vi "cDAQ_PLC.vi"(6 "simulazione":bool, 9 "banco":i32, 11 "carico res":bool=TRUE) -> ()   [LabVIEW 2019]
uses:
  controls/statoDO_Cdaq.ctl
  controls/StatoAO_cdaq.ctl
  cDAQ/SET SINGLE DO.ctl
  cDAQ/DO List.ctl
  cDAQ/SET ARRAY AO.ctl
  cDAQ/SET SINGLE AO.ctl
  cDAQ/AO List.ctl
  TypeDef/Lista AO sistema.ctl
  TypeDef/DOinterfaccia.ctl
  ST1200_LIST_IO/StatoDO_PLC_1.ctl
  ST1200_LIST_IO/StatoDO_PLC_2.ctl
  ST1200_LIST_IO/StatoDO_PLC_3.ctl
  controls/statoAO_plc_1.ctl
  controls/statoAO_plc_2.ctl
  controls/statoAO_plc_3.ctl
  ST1200_LIST_IO/TypeDef_PLC_Q.ctl
  ST1200_LIST_IO/Uscite PLC 2.ctl
  ST1200_LIST_IO/Uscite PLC 3.ctl
  EXIT.vi
  <vilib>/Utility/file.llb/Read Delimited Spreadsheet (string).vi
  Global dati targa SINUSPENTA.vi
panel:
  out "AO Tread ms":u32
  out "DO Tread ms":u32
  out "statoAO_Cdaq out":T1
  out "elements in queue AO":i32
  out "statoDO Cdaq out":T2
  out "elements in queue DO":i32
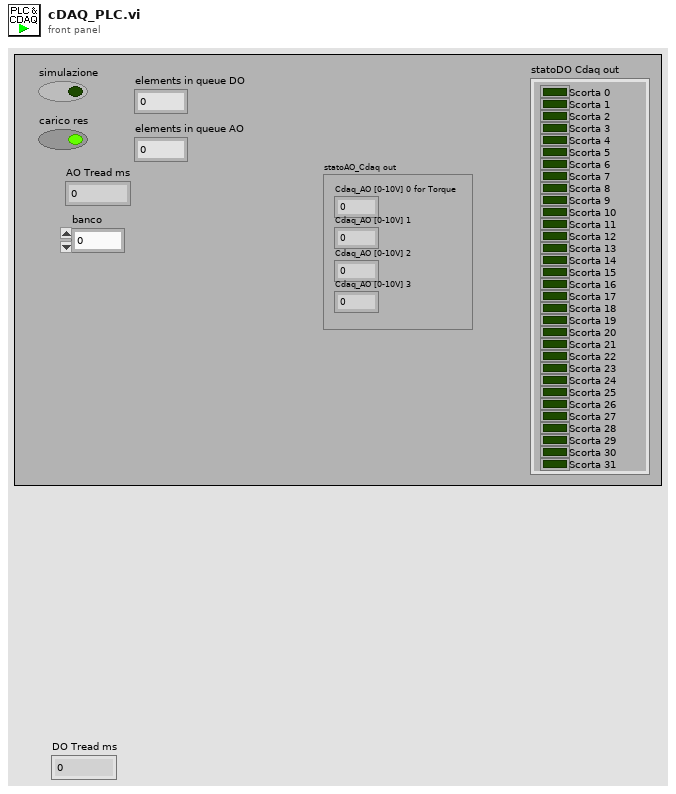
[diagram p1: front panel]
types:
  T1 = typedef "StatoAO_cdaq.ctl" = cluster{"Cdaq_AO [0-10V] 0 for Torque":dbl, "Cdaq_AO [0-10V] 1":dbl, "Cdaq_AO [0-10V] 2":dbl, "Cdaq_AO [0-10V] 3":dbl}
  T2 = typedef "statoDO_Cdaq.ctl" = cluster{"Scorta 0":bool, "Scorta 1":bool, "Scorta 2":bool, "Scorta 3":bool, "Scorta 4":bool, "Scorta 5":bool, "Scorta 6":bool, "Scorta 7":bool, "Scorta 8":bool, "Scorta 9":bool, "Scorta 10":bool, "Scorta 11":bool, "Scorta 12":bool, "Scorta 13":bool, "Scorta 14":bool, "Scorta 15":bool, "Scorta 16":bool, "Scorta 17":bool, "Scorta 18":bool, "Scorta 19":bool, "Scorta 20":bool, "Scorta 21":bool, "Scorta 22":bool, "Scorta 23":bool, "Scorta 24":bool, "Scorta 25":bool, "Scorta 26":bool, "Scorta 27":bool, "Scorta 28":bool, "Scorta 29":bool, "Scorta 30":bool, "Scorta 31":bool}
  T3 = typedef "TypeDef_PLC_Q.ctl" = cluster{"Message":string, "Data":variant}
  T4 = typedef "statoAO_plc_1.ctl" = cluster{"Rif Lim coppia freno [%]":dbl, "Rif rpm freno [%]":dbl, "Rif coppia freno [%]":dbl, "Rif V alimentatore [%]":dbl, "Rif F alimentatore [%]":dbl}
  T5 = typedef "statoAO_plc_2.ctl" = cluster{"Condensatori":dbl, "Scorta 1":dbl, "Scorta 2":dbl}
  T6 = typedef "statoAO_plc_3.ctl" = cluster{"Rif velocità alimentatore":dbl, "Scorta":dbl, "Tipo Motore  keb":dbl, "I nom keb":dbl, "RPM nom keb":dbl, "V nom keb":dbl, "F nom keb":dbl, "t rampa keb":dbl}
  T7 = cluster{"statoAO_PLC 1 in":T4, "statoAO_PLC 2 in":T5, "statoAO_PLC 3 in":T6}
  T8 = typedef "StatoDO_PLC_1.ctl" = cluster{"Scelta banco 1":bool, "Set dati motore freno 2":bool, "Diretto inverter":bool, "Filtro LC":bool, "Marcia ALIM (1s)":bool, "Marcia FRENO (1s)":bool, "Stop AFE (1s)":bool, "Stop freno (1s)":bool, "Reset allarmi":bool, "Watchdog":bool, "Senso rotazione":bool, "Abilita collaudo (1s)":bool, "Disabilita collaudo (1s)":bool, "Abilitazione ALIM":bool, "Abilitazione FRENO":bool, "Teleruttore WT":bool, "Senso rot motore prova":bool, "Scorta 7":bool, "Scorta 8":bool, "Scorta 9":bool, "Scorta 10":bool, "Scorta 11":bool, "Scorta 12":bool, "Scorta 13":bool}
  T9 = typedef "StatoDO_PLC_2.ctl" = cluster{"Relè misura resistomat":bool, "Misura res ramo 1":bool, "Misura res ramo 2":bool, "Misura res ramo 3":bool, "Scelta banco 2":bool, "Scala Torsiometro":bool, "Ctrl torsiometro":bool, "Select current mode":bool, "Select Torque mode":bool, "Select speed mode":bool, "Watchdog":bool, "Scorta":bool, "Scorta 2":bool, "Scorta 3":bool, "Scorta 4":bool, "Scorta 5":bool, "Bench selection":bool, "External alarm":bool, "Enable external program":bool, "Reset allarmi":bool, "Start":bool, "Stop":bool, "Block":bool, "Scorta 6":bool}
  T10 = typedef "StatoDO_PLC_3.ctl" = cluster{"Select linea Inverter":bool, "Abilita sense wattmetro":bool, "Bypass filtro LC":bool, "Filtro LC":bool, "Bypass trasformatore":bool, "Trasformatore":bool, "Abilita uscite variac":bool, "Abilita linea 125 A":bool, "Abilita linea 63 A":bool, "Abilita linea 16 A":bool, "Abilita Scrittura Dati Keb":bool, "Abilita alimentatore":bool, "Marcia alimentatore (1s)":bool, "Stop alimentatore (1s)":bool, "Senso rot mot prova":bool, "Watchdog":bool, "Aumenta tensione variac":bool, "Diminuisci tensione variac ":bool, "Blocco elettroserrature":bool, "Ripristino emergence":bool, "Abilita ingresso variac":bool, "Abilita ventilatore variac":bool, "Reset Allarm":bool, "Scorta 1":bool, "Scorta 2":bool, "Scorta 3":bool, "Scorta 4":bool, "Scorta 5":bool, "Scorta 6":bool, "Scorta 7":bool, "Scorta 8":bool, "Scorta 9":bool, "Abilita collaudo":bool, "Disabilita collaudo ":bool, "Scorta 10":bool, "Scorta 11":bool, "Scorta 12":bool, "Scorta 13":bool, "Scorta 14":bool, "Scorta 15":bool}
  T11 = cluster{"StatoDO_PLC 1 in":T8, "StatoDO_PLC_2_out":T9, "StatoDO_PLC_3_out":T10}
  T12 = typedef "DOinterfaccia.ctl" = cluster{"Scelta banco 1":bool, "Scelta banco 2":bool, "Scelta banco 3":bool, "FRENO 1 abilita":bool, "FRENO 1 start":bool, "FRENO 1 senso rotaz":bool, "FRENO 1 ctrl velocità":bool, "FRENO 2 abilita":bool, "FRENO 2 start":bool, "FRENO 2 senso rotaz":bool, "FRENO 2 ctrl velocità":bool, "ALIM 1 abilita":bool, "ALIM 1 start":bool, "ALIM 2 abilita":bool, "ALIM 2 start":bool, "ALIM 3 abilita":bool, "ALIM 3 start":bool, "Abilita linea trifase":bool, "Abilita linea monofase":bool, "Abilita linea dc":bool, "Abilita linea dc eccit":bool, "B1 Linea elettrica 1":bool, "B1 Linea elettrica 2":bool, "B1 Linea elettrica 3":bool, "B1 Linea elettrica 4":bool, "B1 Linea elettrica 5":bool, "B2 Linea elettrica 1":bool, "B2 Linea elettrica 2":bool, "B2 Linea elettrica 3":bool, "B2 Linea elettrica 4":bool, "B2 Linea elettrica 5":bool, "Start potenza AC":bool, "Stop pontenza AC":bool, "Start potenza DC":bool, "Stop potenza DC":bool, "Start potenza eccitaz":bool, "Stop potenza eccitaz":bool, "Reset allarmi":bool, "watchdog":bool, "Scala torsiometro B1":bool, "Controllo torsiom B1":bool, "Scala torsiometro B2":bool, "Controllo torsiom B2":bool, "Teleruttore WT abilita":bool, "Teleruttore Resistomat abilita":bool, "Teleruttore corto fasi":bool, "Ramo 1 resistomat":bool, "Ramo 2 resistomat":bool, "Ramo 3 resistomat":bool, "Collaudo in corso":bool, "Allarme presente":bool, "Enable Res Meter":bool, "Bypass Res Meter":bool, "2nd canale Res Meter":bool, "Scala 200/2000 res meter":bool, "Taratura res meter":bool, "FRENO 1 ctrl coppia":bool, "FRENO 2 ctrl coppia":bool, "FRENO 3 ctrl coppia":bool, "Aggiuntivi impianto":cluster{"Senso rotazione alim 1":bool, "Senso rotazione alim 2":bool}, "ALIM 1 stop":bool, "ALIM 2 stop":bool, "ALIM 3 stop":bool, "FRENO 1 stop":bool, "FRENO 2 stop":bool, "FRENO 3 stop":bool, "B1 configurazione freno B":bool, "B2 configurazione freno B":bool, "Abilita scrittura KEB":bool, "Bench Selection (0-B1,1-B2)":bool, "Select current mode":bool, "Select torque mode":bool, "Select speed mode":bool, "Start":bool, "Stop":bool, "Block":bool, "Enable Force mode":bool, "Abilita linea 125 A":bool, "Abilita linea 63 A":bool, "Abilita linea 16 A":bool, "Aum Tensione Variac":bool, "Dim Tesnione Variac":bool, "Abilita ellectro stractura":bool, "Risprinito Emergence":bool, "Abilita collaudo":bool, "Disabilita collaudo":bool, "External Alaram":bool, "Enable external program":bool, "Reset":bool, "Abilita Ingresso Variac":bool, "Abilita Ventilatore Variac":bool, "Abilita Uscita Variac ":bool}
  T13 = typedef "Lista AO sistema.ctl" = cluster{"FRENO1 rif vel":dbl, "FRENO1 rif Coppia":dbl, "FRENO2 rif vel":dbl, "FRENO2 rif Coppia":dbl, "ALIM1 rif V":dbl, "ALIM1 rif F":dbl, "ALIM2 rif V":dbl, "ALIM2 rif F":dbl, "ALIM3 rif V":dbl, "ALIM3 rif F":dbl, "Fnom keb":dbl, "Rpm nom keb":dbl, "Pnom keb":dbl, "Inom keb":dbl, "Vnom keb":dbl, "Rpm max keb":dbl, "Tempo rampa keb":dbl, "Tipo Mot keb":dbl, "FRENO  rif Coppia ":dbl, "FRENO  rif  Corrente":dbl}
  T14 = typedef "SET ARRAY AO.ctl" = T15[]
  T15 = typedef "SET SINGLE AO.ctl" = cluster{"AO":T16, "Value":dbl}
  T16 = typedef "AO List.ctl" = enum16{"OFF: ALL AO", "RIF VEL FRENO 1", "RIF VEL FRENO 2", "RIF VEL FRENO 3", "RIF COPPIA FRENO", "RIF COPPIA FRENO 1", "RIF COPPIA FRENO 2", "RIF COPPIA FRENO 3", "RIF CORRENTE FRENO 2", "RIF V ALIM 1", "RIF F ALIM 1", "RIF V ALIM 2", "RIF F ALIM 2", "RIF V ALIM 3", "RIF F ALIM 3", "RIF V ALIM 4", "RIF F ALIM 4", "FORZA AO PLC 3", "FORZA AO PLC 2", "FORZA AO PLC 1", "FORZA AO cDAQ", "Configura alimentatore keb", "Tempo rampa keb", "Condensatori", "Exit"}
  T17 = typedef "SET SINGLE DO.ctl" = cluster{"DO":T18, "Value":bool}
  T18 = typedef "DO List.ctl" = enum16{"OFF: ALL DO", "*ABILITA freno 1", "*ABILITA freno 2", "*ABILITA freno 3", "*START freno 1", "*START freno 2", "*START freno 3", "*STOP freno 1", "*STOP freno 3", "*STOP freno 2", "*Senso rot freno 1", "*Senso rot freno 2", "*Senso rot freno 3", "*Ctrl velocità freno 1", "*Ctrl velocità freno 2", "*Ctrl velocità freno 3", "*Ctrl coppia freno 1", "*Ctrl coppia freno 2", "*Ctrl coppia freno 3", "*ABILITA alimentatore 1", "*ABILITA alimentatore 2", "*ABILITA alimentatore 3", "*ABILITA alimentatore 4", "*START alimentatore 1", "*START alimentatore 2", "*START alimentatore 3", "*START alimentatore 4", "*STOP alimentatore 1", "*STOP alimentatore 2", "*STOP alimentatore 3", "*STOP alimentatore 4", "SENSO ROT alimentatore 1", "SENSO ROT alimentatore 2", "Abilita LEM 1000A", "Abilita LEM 300A", "Abilita sensori EXT WT", "B1 Seleziona linea 1", "B1 Seleziona linea 2", "B1 Seleziona linea 3", "B1 Seleziona linea 4", "B1 Seleziona linea 5", "B2 Seleziona linea 1", "B2 Seleziona linea 2", "B2 Seleziona linea 3", "B2 Seleziona linea 4", "B2 Seleziona linea 5", "*Reset allarmi", "*Start potenza AC", "*Stop potenza AC", "*Start potenza DC", "*Stop potenza DC", "*Start potenza DC eccit", "*Stop pontenza DC eccit", "Bypass res meter", "2nd canale res meter", "Enable res meter", "*Abilit teler ramo WT", "*Abil teler ramo princ Resit", "*Abil teler ramo 1 Resist", "*Abil teler ramo 2 Resist", "*Abil teler ramo 3 Resist", "*Abil cortocirc avvolgim", "*Controllo torsiometro B1", "*Controllo Torsiom B2", "*Scala torsiometro B1", "*Scala torsiometro B2", "*Collaudo in corso", "*Allarme presente", "Abilitazione elettroserratura", "Exit", "*Abilita collaudo", "*Abilita potenza trifase", "*Abilita potenza monofase", "*Abilita potenza DC", "*Abilita potenza DC eccit", "*Disabilita teleruttori potenza", "Set teleruttori prova a freddo", "Prova a freddo monofase", "Watchdog", "Forza DO PLC 3", "Forza DO PLC 2", "Forza DO PLC 1", "Forza DO cDAQ", "Scala 2000(T) 200(F) res meter", "Seleziona banco 1", "Seleziona banco 2", "Comando azionam in blocco", "Comando azionam reset", "Sensibilità freno 16 32 nm", "Reset Allarmi", "Carico res - Ramo 1", "Carico res - Ramo 2", "Carico res - Ramo 3", "Carico res - Ramo 4", "Carico res - Ramo 5", "Carico res - Ramo 6", "Carico res - Ramo 7", "Carico res - Ramo 8", "Carico res - Ramo 9", "Carico res - Ramo 10", "Carico res - Ramo 11", "Carico res - Start ventilatore", "Carico res - Stop ventilatore", "Abilita potenza solo freno", "Abilita AFE + freno trasc", "Abilita potenza carico resistivo", "Chiudi potenza AFE", "Apri potenza AFE", "Start AFE", "Config Banco2 TDE", "Misura diretto WT", "Ripristina centralina protezioni", "Abilita Scrittura Dati Keb", "Bench Selection(0-B1,1-B2)", "Select current mode", "Select torque mode", "Select speed mode", "Extenal alarm", "Enable Extenal program ", "Start ", "Stop", "Enable force mode", "Abilita linea 125 A", "Abilita linea 63 A", "Abilita linea 16 A", "Aum Tensione Variac", "Dim Tesnione Variac", "Abilita Ellecto Stractura", "Riprinto Emergenxe ", "Abilita Collaudo", "Disabilita Collaudo", "Abilita Ingresso Variac", "Abilita Uscita Variac", "Abilita ventilatore Variac"}
  T19 = typedef "Uscite PLC 2.ctl" = cluster{"AO (real) 2":cluster{"SCORTA 1":dbl, "SCORTA 2":dbl, "SCORTA 3":dbl, "SCORTA 4":dbl, "SCORTA 5":dbl, "SCORTA 6":dbl, "SCORTA 7":dbl, "SCORTA 8":dbl}, "statoAO_PLC out":T5, "DO (bit)":T9}
  T20 = typedef "Uscite PLC 3.ctl" = cluster{"AO (real) 2":cluster{"SCORTA 1":dbl, "SCORTA 2":dbl, "SCORTA 3":dbl, "SCORTA 4":dbl, "SCORTA 5":dbl, "SCORTA 6":dbl, "SCORTA 7":dbl, "SCORTA 8":dbl}, "statoAO_PLC out":T6, "DO (bit)":T10}
  T21 = cluster{"StatoDO_PLC 1":T8, "StatoDO_PLC_2":T9, "StatoDO_PLC_3":T10}
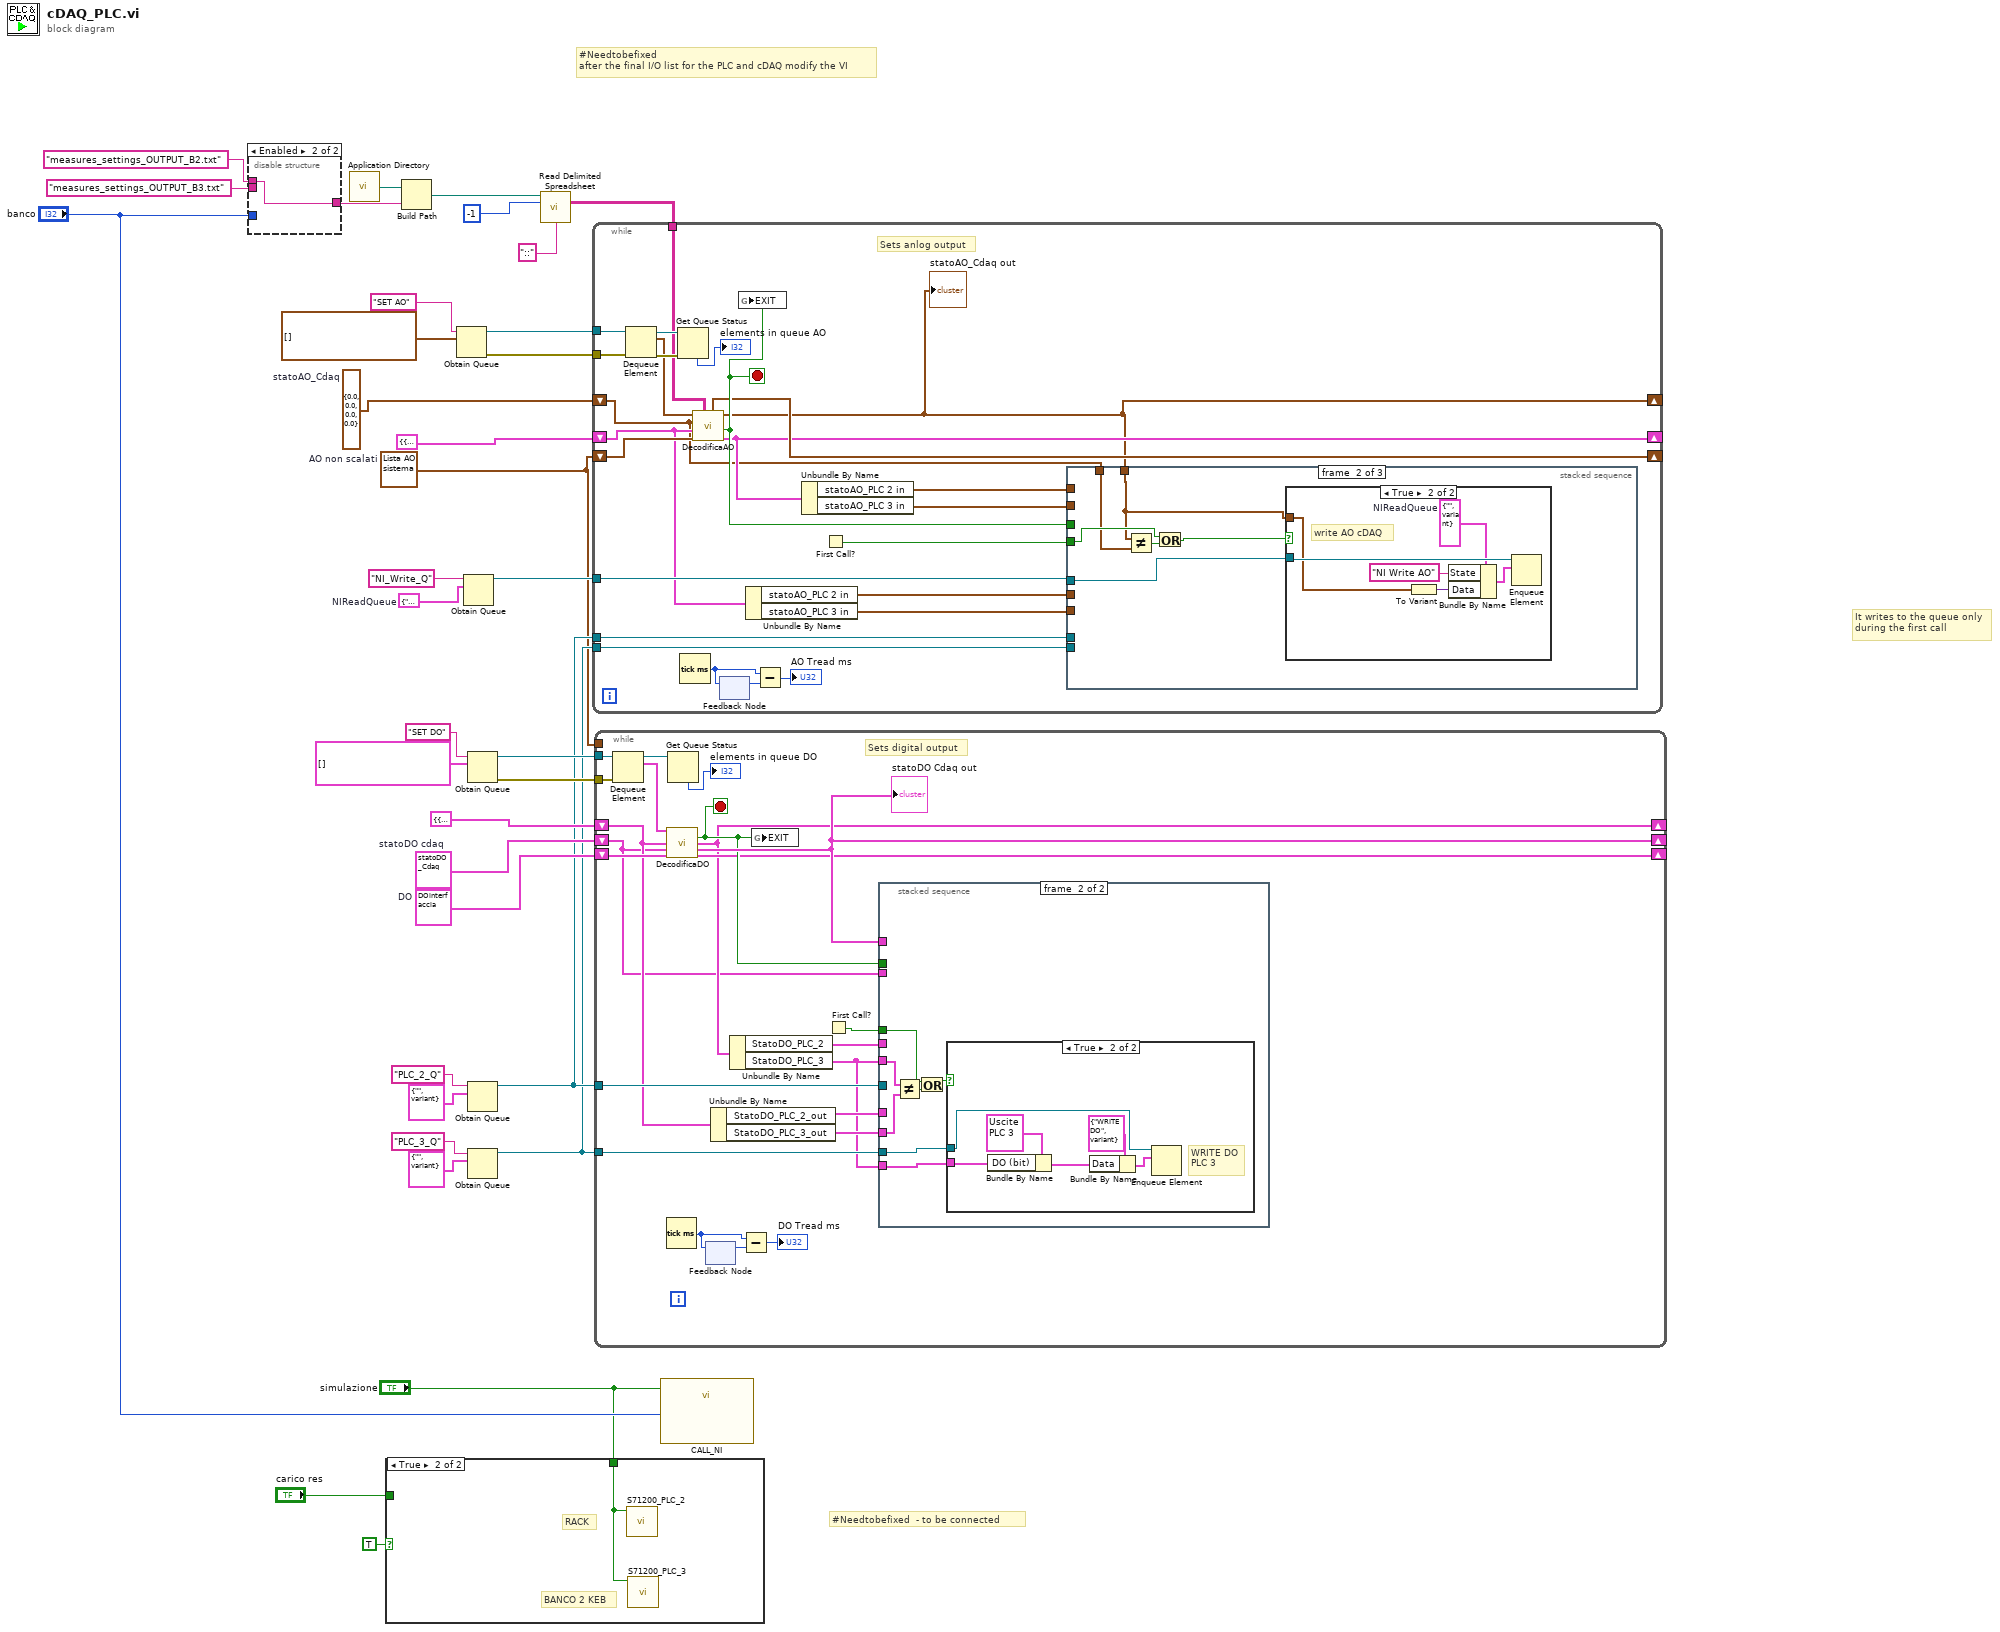
[diagram p0: block diagram]
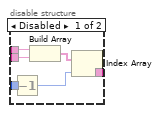
[diagram p2: hidden frame]
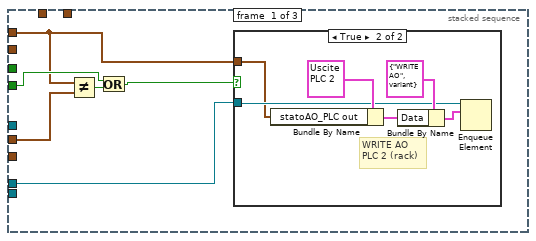
[diagram p4: hidden frame]
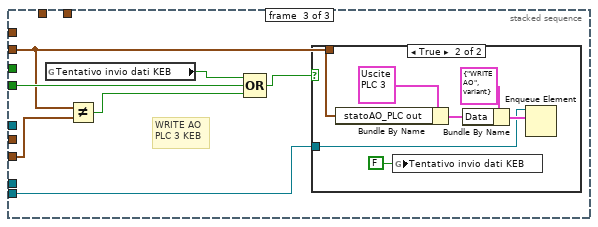
[diagram p7: hidden frame]
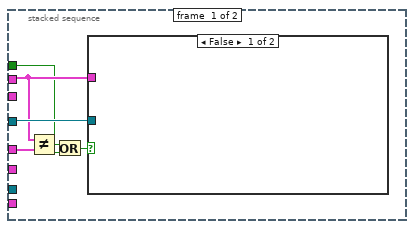
[diagram p9: hidden frame]
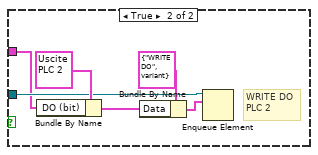
[diagram p10: hidden frame]
diagram:
  w3 = cluster{string, variant} {"", variant}  # NIReadQueue
  w24 = T12 {"Scelta banco 1"=FALSE, "Scelta banco 2"=FALSE, "Scelta banco 3"=FALSE, "FRENO 1 abilita"=FALSE, "FRENO 1 start"=FALSE, "FRENO 1 senso rotaz"=FALSE, "FRENO 1 ctrl velocità"=FALSE, "FRENO 2 abilita"=FALSE, "FRENO 2 start"=FALSE, "FRENO 2 senso rotaz"=FALSE, "FRENO 2 ctrl velocità"=FALSE, "ALIM 1 abilita"=FALSE, "ALIM 1 start"=FALSE, "ALIM 2 abilita"=FALSE, "ALIM 2 start"=FALSE, "ALIM 3 abilita"=FALSE, "ALIM 3 start"=FALSE, "Abilita linea trifase"=FALSE, "Abilita linea monofase"=FALSE, "Abilita linea dc"=FALSE, "Abilita linea dc eccit"=FALSE, "B1 Linea elettrica 1"=FALSE, "B1 Linea elettrica 2"=FALSE, "B1 Linea elettrica 3"=FALSE, "B1 Linea elettrica 4"=FALSE, "B1 Linea elettrica 5"=FALSE, "B2 Linea elettrica 1"=FALSE, "B2 Linea elettrica 2"=FALSE, "B2 Linea elettrica 3"=FALSE, "B2 Linea elettrica 4"=FALSE, "B2 Linea elettrica 5"=FALSE, "Start potenza AC"=FALSE, "Stop pontenza AC"=FALSE, "Start potenza DC"=FALSE, "Stop potenza DC"=FALSE, "Start potenza eccitaz"=FALSE, "Stop potenza eccitaz"=FALSE, "Reset allarmi"=FALSE, "watchdog"=FALSE, "Scala torsiometro B1"=FALSE, "Controllo torsiom B1"=FALSE, "Scala torsiometro B2"=FALSE, "Controllo torsiom B2"=FALSE, "Teleruttore WT abilita"=FALSE, "Teleruttore Resistomat abilita"=FALSE, "Teleruttore corto fasi"=FALSE, "Ramo 1 resistomat"=FALSE, "Ramo 2 resistomat"=FALSE, "Ramo 3 resistomat"=FALSE, "Collaudo in corso"=FALSE, "Allarme presente"=FALSE, "Enable Res Meter"=FALSE, "Bypass Res Meter"=FALSE, "2nd canale Res Meter"=FALSE, "Scala 200/2000 res meter"=FALSE, "Taratura res meter"=FALSE, "FRENO 1 ctrl coppia"=FALSE, "FRENO 2 ctrl coppia"=FALSE, "FRENO 3 ctrl coppia"=FALSE, "Aggiuntivi impianto"={"Senso rotazione alim 1"=FALSE, "Senso rotazione alim 2"=FALSE}, "ALIM 1 stop"=FALSE, "ALIM 2 stop"=FALSE, "ALIM 3 stop"=FALSE, "FRENO 1 stop"=FALSE, "FRENO 2 stop"=FALSE, "FRENO 3 stop"=FALSE, "B1 configurazione freno B"=FALSE, "B2 configurazione freno B"=FALSE, "Abilita scrittura KEB"=FALSE, "Bench Selection (0-B1,1-B2)"=FALSE, "Select current mode"=FALSE, "Select torque mode"=FALSE, "Select speed mode"=FALSE, "Start"=FALSE, "Stop"=FALSE, "Block"=FALSE, "Enable Force mode"=FALSE, "Abilita linea 125 A"=FALSE, "Abilita linea 63 A"=FALSE, "Abilita linea 16 A"=FALSE, "Aum Tensione Variac"=FALSE, "Dim Tesnione Variac"=FALSE, "Abilita ellectro stractura"=FALSE, "Risprinito Emergence"=FALSE, "Abilita collaudo"=FALSE, "Disabilita collaudo"=FALSE, "External Alaram"=FALSE, "Enable external program"=FALSE, "Reset"=FALSE, "Abilita Ingresso Variac"=FALSE, "Abilita Ventilatore Variac"=FALSE, "Abilita Uscita Variac "=FALSE}  # DO
  w4 = T13 {"FRENO1 rif vel"=0.0, "FRENO1 rif Coppia"=0.0, "FRENO2 rif vel"=0.0, "FRENO2 rif Coppia"=0.0, "ALIM1 rif V"=0.0, "ALIM1 rif F"=0.0, "ALIM2 rif V"=0.0, "ALIM2 rif F"=0.0, "ALIM3 rif V"=0.0, "ALIM3 rif F"=0.0, "Fnom keb"=0.0, "Rpm nom keb"=0.0, "Pnom keb"=0.0, "Inom keb"=0.0, "Vnom keb"=0.0, "Rpm max keb"=0.0, "Tempo rampa keb"=0.0, "Tipo Mot keb"=0.0, "FRENO  rif Coppia "=0.0, "FRENO  rif  Corrente"=0.0}  # AO non scalati
  w2 = T1 {"Cdaq_AO [0-10V] 0 for Torque"=0.0, "Cdaq_AO [0-10V] 1"=0.0, "Cdaq_AO [0-10V] 2"=0.0, "Cdaq_AO [0-10V] 3"=0.0}  # statoAO_Cdaq
  w35 = T2 {"Scorta 0"=FALSE, "Scorta 1"=FALSE, "Scorta 2"=FALSE, "Scorta 3"=FALSE, "Scorta 4"=FALSE, "Scorta 5"=FALSE, "Scorta 6"=FALSE, "Scorta 7"=FALSE, "Scorta 8"=FALSE, "Scorta 9"=FALSE, "Scorta 10"=FALSE, "Scorta 11"=FALSE, "Scorta 12"=FALSE, "Scorta 13"=FALSE, "Scorta 14"=FALSE, "Scorta 15"=FALSE, "Scorta 16"=FALSE, "Scorta 17"=FALSE, "Scorta 18"=FALSE, "Scorta 19"=FALSE, "Scorta 20"=FALSE, "Scorta 21"=FALSE, "Scorta 22"=FALSE, "Scorta 23"=FALSE, "Scorta 24"=FALSE, "Scorta 25"=FALSE, "Scorta 26"=FALSE, "Scorta 27"=FALSE, "Scorta 28"=FALSE, "Scorta 29"=FALSE, "Scorta 30"=FALSE, "Scorta 31"=FALSE}  # statoDO cdaq
  # "#Needtobefixed\nafter the final I/O list for the PLC and cDAQ modify the VI"
  # "It writes to the queue only\nduring the first call"
  # "#Needtobefixed  - to be connected"
  n1 = disable-structure shown="Enabled" {
    disable-tunnel: "measures_settings_OUTPUT_B2.txt" ("name or relative path") -> [w41 w42]
    disable-tunnel: "measures_settings_OUTPUT_B3.txt" ("name or relative path") -> [w40 _]
    disable-tunnel: [w37 w42] -> w16
    disable-tunnel: "banco" -> [w36 _]
    frame Disabled {
      n2 = Decrement(x=w36) -> (x-1=w38:i32)
      n3 = Build Array(w41, w40) -> (w39:string[])
      n4 = Index Array(array=w39, index=w38) -> (element=w37:string)
    }
    frame Enabled {
    }
  }
  n5 = call <vilib>:"Application Directory.vi"() -> ("Application Directory"=w23:path)
  n6 = case shown="True" TRUE {
    tunnel: "simulazione" -> [_ w43]
    tunnel: "carico res" -> [_ _]
    frame False {
    }
    frame True {
      # "BANCO 2 KEB"
      # "RACK"
      n7 = call "S71200_PLC_2.vi"("Simulazione"=w43) -> ()  [unwired: 11 in]
      n8 = call "S71200_PLC_3.vi"("Simulazione"=w43) -> ()  [unwired: 11 in]
    }
  }
  n9 = Build Path(base path=w23, name or relative path=w16) -> (appended path=w22:path)
  n10 = Obtain Queue(name (unnamed)="SET AO", element data type=T14 [] ("Cluster SET AO")) -> (queue out=w29:refnum<queue>, error out=w28:errorcluster)  [unwired: 3 in, 1 out]
  n11 = Obtain Queue(name (unnamed)="NI_Write_Q", element data type=w3) -> (queue out=w26:refnum<queue>)  [unwired: 3 in, 2 out]
  n12 = Obtain Queue(name (unnamed)="SET DO", element data type=T17[] []) -> (queue out=w34:refnum<queue>, error out=w33:errorcluster)  [unwired: 3 in, 1 out]
  n13 = Obtain Queue(name (unnamed)="PLC_2_Q", element data type=T3 {"Message"="", "Data"=variant}) -> (queue out=w7:refnum<queue>)  [unwired: 3 in, 2 out]
  n14 = Obtain Queue(name (unnamed)="PLC_3_Q", element data type=T3 {"Message"="", "Data"=variant}) -> (queue out=w6:refnum<queue>)  [unwired: 3 in, 2 out]
  n15 = call-poly <vilib>:"Read Delimited Spreadsheet.vi"("file path (dialog if empty)"=w22, "number of rows (all:-1)"=-1, "delimiter (\\t)"="::" ("delimiter (\\t)")) -> ("all rows"=w19:string[][])  [unwired: 7 in, 5 out]
  n16 = while {
    tunnel: w29 -> [w68]
    tunnel: w28 -> [w67]
    shift-right: [w57] -> _
    shift-left: T7 {"statoAO_PLC 1 in"={"Rif Lim coppia freno [%]"=0.0, "Rif rpm freno [%]"=0.0, "Rif coppia freno [%]"=0.0, "Rif V alimentatore [%]"=0.0, "Rif F alimentatore [%]"=0.0}, "statoAO_PLC 2 in"={"Condensatori"=0.0, "Scorta 1"=0.0, "Scorta 2"=0.0}, "statoAO_PLC 3 in"={"Rif velocità alimentatore"=0.0, "Scorta"=0.0, "Tipo Motore  keb"=0.0, "I nom keb"=0.0, "RPM nom keb"=0.0, "V nom keb"=0.0, "F nom keb"=0.0, "t rampa keb"=0.0}} ("AO PLCs out") -> [w51]
    tunnel: w26 -> [w63]
    shift-right: [w60] -> _
    shift-left: w4 -> [w59]
    tunnel: w19 -> [w58]
    tunnel: w7 -> [w54]
    tunnel: w6 -> [w53]
    shift-right: [w48] -> _
    shift-left: w2 -> [w47]
    stop <- w61 stop-if-true
    # "Sets anlog output"
    n17 = Dequeue Element(queue=w68, error in (no error)=w67) -> (queue out=w65:refnum<queue>, element=w64:T14, error out=w66:errorcluster)  [unwired: 1 in, 1 out]
    n18 = Get Queue Status(queue=w65, error in (no error)=w66) -> (# elements in queue=→"elements in queue AO":i32)  [unwired: 1 in, 7 out]
    n19 = Tick Count (ms)() -> (millisecond timer value=w44:u32)
    n20 = call "DecodificaAO.vi"("Caratteristiche Caricate"=w58, "AO non scalati IN"=w59, "AO PLCs in"=w51, "statoAO_Cdaq in"=w47, "Cluster SET AO"=w64) -> ("AO PLCs out"=w57:T7, "exit"=w61:bool, "statoAO_Cdaq out"=w48:T1, "AO non scalati OUT"=w60:T13)  [unwired: 3 in]
    "statoAO_Cdaq out" <- w48
    n21 = feedback #1() -> (w45:u32)  [unwired: 1 in]
    n22 = feedback-in #1(w44) -> ()
    n23 = global write "EXIT.vi" "EXIT"(w61) -> ()
    n24 = Unbundle By Name(w51) -> ("statoAO_PLC 2 in"=w50:T5, "statoAO_PLC 3 in"=w49:T6)
    n25 = Subtract(x=w44, y=w45) -> (x-y=→"AO Tread ms":u32)
    n26 = Unbundle By Name(w57) -> ("statoAO_PLC 2 in"=w56:T5, "statoAO_PLC 3 in"=w55:T6)
    n27 = First Call?() -> (First Call?: T/F=w52:bool)
    n28 = stacked-sequence {
      tunnel: w63 -> [_ w83 _]
      tunnel: w48 -> [_ w82 _]
      tunnel: w61 -> [_ _ _]
      tunnel: w56 -> [w70 _ _]
      tunnel: w55 -> [_ _ w94]
      tunnel: w54 -> [w74 _ _]
      tunnel: w53 -> [_ _ w99]
      tunnel: w52 -> [w73 w86 w98]
      tunnel: w50 -> [w71 _ _]
      tunnel: w49 -> [_ _ w95]
      tunnel: w47 -> [_ w81 _]
      frame #0 {
        n29 = Not Equal?(x=w70, y=w71) -> (x != y?=w69:bool)
        n30 = Or(x=w73, y=w69) -> (x .or. y?=w72:bool)
        n31 = case shown="True" w72 {
          tunnel: w74 -> [_ w76]
          tunnel: w70 -> [_ w75]
          frame False {
          }
          frame True {
            # "WRITE AO\nPLC 2 (rack)"
            n32 = Bundle By Name(cluster=T19 {"AO (real) 2"={"SCORTA 1"=0.0, "SCORTA 2"=0.0, "SCORTA 3"=0.0, "SCORTA 4"=0.0, "SCORTA 5"=0.0, "SCORTA 6"=0.0, "SCORTA 7"=0.0, "SCORTA 8"=0.0}, "statoAO_PLC out"={"Condensatori"=0.0, "Scorta 1"=0.0, "Scorta 2"=0.0}, "DO (bit)"={"Relè misura resistomat"=FALSE, "Misura res ramo 1"=FALSE, "Misura res ramo 2"=FALSE, "Misura res ramo 3"=FALSE, "Scelta banco 2"=FALSE, "Scala Torsiometro"=FALSE, "Ctrl torsiometro"=FALSE, "Select current mode"=FALSE, "Select Torque mode"=FALSE, "Select speed mode"=FALSE, "Watchdog"=FALSE, "Scorta"=FALSE, "Scorta 2"=FALSE, "Scorta 3"=FALSE, "Scorta 4"=FALSE, "Scorta 5"=FALSE, "Bench selection"=FALSE, "External alarm"=FALSE, "Enable external program"=FALSE, "Reset allarmi"=FALSE, "Start"=FALSE, "Stop"=FALSE, "Block"=FALSE, "Scorta 6"=FALSE}} ("USCITE PLC"), "statoAO_PLC out"=w75) -> (w80:T19)
            n33 = Bundle By Name(cluster=T3 {"Message"="WRITE AO", "Data"=variant}, "Data"=w80) -> (w78:T3)
            n34 = Enqueue Element(queue=w76, element=w78) -> ()  [unwired: 2 in, 3 out]
          }
        }
      }
      frame #1 {
        n35 = Not Equal?(x=w82, y=w81) -> (x != y?=w84:bool)
        n36 = Or(x=w86, y=w84) -> (x .or. y?=w85:bool)
        n37 = case shown="True" w85 {
          tunnel: w83 -> [_ w92]
          tunnel: w82 -> [_ w89]
          frame False {
          }
          frame True {
            w91 = cluster{"State":string, "Data":variant} {"State"="", "Data"=variant}  # NIReadQueue
            # "write AO cDAQ"
            n38 = To Variant(anything=w89) -> (Variant=w90:variant)
            n39 = Bundle By Name(cluster=w91, "State"="NI Write AO", "Data"=w90) -> (w87:cluster{"State":string, "Data":variant})
            n40 = Enqueue Element(queue=w92, element=w87) -> ()  [unwired: 2 in, 3 out]
          }
        }
      }
      frame #2 {
        # "WRITE AO\nPLC 3 KEB"
        n41 = global read "Global dati targa SINUSPENTA.vi" "Tentativo invio dati KEB"() -> (w96:bool)
        n42 = Not Equal?(x=w94, y=w95) -> (x != y?=w93:bool)
        n43 = Compound Arithmetic op=OR(w96, w98, w93) -> (w97:bool)
        n44 = case shown="True" w97 {
          tunnel: w99 -> [_ w102]
          tunnel: w94 -> [_ w101]
          frame False {
          }
          frame True {
            n45 = Bundle By Name(cluster=T20 {"AO (real) 2"={"SCORTA 1"=0.0, "SCORTA 2"=0.0, "SCORTA 3"=0.0, "SCORTA 4"=0.0, "SCORTA 5"=0.0, "SCORTA 6"=0.0, "SCORTA 7"=0.0, "SCORTA 8"=0.0}, "statoAO_PLC out"={"Rif velocità alimentatore"=0.0, "Scorta"=0.0, "Tipo Motore  keb"=0.0, "I nom keb"=0.0, "RPM nom keb"=0.0, "V nom keb"=0.0, "F nom keb"=0.0, "t rampa keb"=0.0}, "DO (bit)"={"Select linea Inverter"=FALSE, "Abilita sense wattmetro"=FALSE, "Bypass filtro LC"=FALSE, "Filtro LC"=FALSE, "Bypass trasformatore"=FALSE, "Trasformatore"=FALSE, "Abilita uscite variac"=FALSE, "Abilita linea 125 A"=FALSE, "Abilita linea 63 A"=FALSE, "Abilita linea 16 A"=FALSE, "Abilita Scrittura Dati Keb"=FALSE, "Abilita alimentatore"=FALSE, "Marcia alimentatore (1s)"=FALSE, "Stop alimentatore (1s)"=FALSE, "Senso rot mot prova"=FALSE, "Watchdog"=FALSE, "Aumenta tensione variac"=FALSE, "Diminuisci tensione variac "=FALSE, "Blocco elettroserrature"=FALSE, "Ripristino emergence"=FALSE, "Abilita ingresso variac"=FALSE, "Abilita ventilatore variac"=FALSE, "Reset Allarm"=FALSE, "Scorta 1"=FALSE, "Scorta 2"=FALSE, "Scorta 3"=FALSE, "Scorta 4"=FALSE, "Scorta 5"=FALSE, "Scorta 6"=FALSE, "Scorta 7"=FALSE, "Scorta 8"=FALSE, "Scorta 9"=FALSE, "Abilita collaudo"=FALSE, "Disabilita collaudo "=FALSE, "Scorta 10"=FALSE, "Scorta 11"=FALSE, "Scorta 12"=FALSE, "Scorta 13"=FALSE, "Scorta 14"=FALSE, "Scorta 15"=FALSE}} ("USCITE PLC"), "statoAO_PLC out"=w101) -> (w104:T20)
            n46 = global write "Global dati targa SINUSPENTA.vi" "Tentativo invio dati KEB"(FALSE ("Tentativo invio dati KEB")) -> ()
            n47 = Bundle By Name(cluster=T3 {"Message"="WRITE AO", "Data"=variant}, "Data"=w104) -> (w103:T3)
            n48 = Enqueue Element(queue=w102, element=w103) -> ()  [unwired: 2 in, 3 out]
          }
        }
      }
    }
  }
  n49 = while {
    tunnel: w34 -> [w127]
    tunnel: w33 -> [w128]
    shift-right: [w124] -> _
    shift-left: w35 -> [w114]
    shift-right: [w119] -> _
    shift-left: T11 {"StatoDO_PLC 1 in"={"Scelta banco 1"=FALSE, "Set dati motore freno 2"=FALSE, "Diretto inverter"=FALSE, "Filtro LC"=FALSE, "Marcia ALIM (1s)"=FALSE, "Marcia FRENO (1s)"=FALSE, "Stop AFE (1s)"=FALSE, "Stop freno (1s)"=FALSE, "Reset allarmi"=FALSE, "Watchdog"=FALSE, "Senso rotazione"=FALSE, "Abilita collaudo (1s)"=FALSE, "Disabilita collaudo (1s)"=FALSE, "Abilitazione ALIM"=FALSE, "Abilitazione FRENO"=FALSE, "Teleruttore WT"=FALSE, "Senso rot motore prova"=FALSE, "Scorta 7"=FALSE, "Scorta 8"=FALSE, "Scorta 9"=FALSE, "Scorta 10"=FALSE, "Scorta 11"=FALSE, "Scorta 12"=FALSE, "Scorta 13"=FALSE}, "StatoDO_PLC_2_out"={"Relè misura resistomat"=FALSE, "Misura res ramo 1"=FALSE, "Misura res ramo 2"=FALSE, "Misura res ramo 3"=FALSE, "Scelta banco 2"=FALSE, "Scala Torsiometro"=FALSE, "Ctrl torsiometro"=FALSE, "Select current mode"=FALSE, "Select Torque mode"=FALSE, "Select speed mode"=FALSE, "Watchdog"=FALSE, "Scorta"=FALSE, "Scorta 2"=FALSE, "Scorta 3"=FALSE, "Scorta 4"=FALSE, "Scorta 5"=FALSE, "Bench selection"=FALSE, "External alarm"=FALSE, "Enable external program"=FALSE, "Reset allarmi"=FALSE, "Start"=FALSE, "Stop"=FALSE, "Block"=FALSE, "Scorta 6"=FALSE}, "StatoDO_PLC_3_out"={"Select linea Inverter"=FALSE, "Abilita sense wattmetro"=FALSE, "Bypass filtro LC"=FALSE, "Filtro LC"=FALSE, "Bypass trasformatore"=FALSE, "Trasformatore"=FALSE, "Abilita uscite variac"=FALSE, "Abilita linea 125 A"=FALSE, "Abilita linea 63 A"=FALSE, "Abilita linea 16 A"=FALSE, "Abilita Scrittura Dati Keb"=FALSE, "Abilita alimentatore"=FALSE, "Marcia alimentatore (1s)"=FALSE, "Stop alimentatore (1s)"=FALSE, "Senso rot mot prova"=FALSE, "Watchdog"=FALSE, "Aumenta tensione variac"=FALSE, "Diminuisci tensione variac "=FALSE, "Blocco elettroserrature"=FALSE, "Ripristino emergence"=FALSE, "Abilita ingresso variac"=FALSE, "Abilita ventilatore variac"=FALSE, "Reset Allarm"=FALSE, "Scorta 1"=FALSE, "Scorta 2"=FALSE, "Scorta 3"=FALSE, "Scorta 4"=FALSE, "Scorta 5"=FALSE, "Scorta 6"=FALSE, "Scorta 7"=FALSE, "Scorta 8"=FALSE, "Scorta 9"=FALSE, "Abilita collaudo"=FALSE, "Disabilita collaudo "=FALSE, "Scorta 10"=FALSE, "Scorta 11"=FALSE, "Scorta 12"=FALSE, "Scorta 13"=FALSE, "Scorta 14"=FALSE, "Scorta 15"=FALSE}} ("DO PLCs out") -> [w115]
    shift-right: [w121] -> _
    shift-left: w24 -> [w120]
    tunnel: w7 -> [w117]
    tunnel: w6 -> [w116]
    tunnel: w4 -> [_]
    stop <- w122 stop-if-true
    # "Sets digital output"
    n50 = Dequeue Element(queue=w127, error in (no error)=w128) -> (queue out=w125:refnum<queue>, element=w126:T17[])  [unwired: 1 in, 2 out]
    n51 = Tick Count (ms)() -> (millisecond timer value=w109:u32)
    n52 = call "DecodificaDO.vi"("Array"=w126, "DO PLCs in"=w115, "statoDO Cdaq in"=w114, "DO interfaccia in"=w120) -> ("Exit?"=w122:bool, "DO PLCs out"=w119:T21, "statoDO Cdaq out"=w124:T2, "DO interfaccia out"=w121:T12)  [unwired: 8 in]
    "statoDO Cdaq out" <- w124
    n53 = Get Queue Status(queue=w125) -> (# elements in queue=→"elements in queue DO":i32)  [unwired: 2 in, 7 out]
    n54 = feedback #2() -> (w108:u32)  [unwired: 1 in]
    n55 = feedback-in #2(w109) -> ()
    n56 = Unbundle By Name(w115) -> ("StatoDO_PLC_2_out"=w113:T9, "StatoDO_PLC_3_out"=w112:T10)
    n57 = Unbundle By Name(w119) -> ("StatoDO_PLC_2"=w118:T9, "StatoDO_PLC_3"=w111:T10)
    n58 = Subtract(x=w109, y=w108) -> (x-y=→"DO Tread ms":u32)
    n59 = global write "EXIT.vi" "EXIT"(w122) -> ()
    n60 = First Call?() -> (First Call?: T/F=w110:bool)
    n61 = stacked-sequence {
      tunnel: w124 -> [_ _]
      tunnel: w122 -> [_ _]
      tunnel: w118 -> [w133 _]
      tunnel: w111 -> [_ w146]
      tunnel: w117 -> [w134 _]
      tunnel: w116 -> [_ w147]
      tunnel: w114 -> [_ _]
      tunnel: w113 -> [w132 _]
      tunnel: w112 -> [_ w145]
      tunnel: w111 -> [_ w144]
      tunnel: w110 -> [w129 w141]
      frame #0 {
        n62 = Not Equal?(x=w133, y=w132) -> (x != y?=w131:bool)
        n63 = Or(x=w131, y=w129) -> (x .or. y?=w130:bool)
        n64 = case shown="False" w130 {
          tunnel: w134 -> [_ w136]
          tunnel: w133 -> [_ w135]
          frame False {
          }
          frame True {
            # "WRITE DO\nPLC 2"
            n65 = Bundle By Name(cluster=T19 {"AO (real) 2"={"SCORTA 1"=0.0, "SCORTA 2"=0.0, "SCORTA 3"=0.0, "SCORTA 4"=0.0, "SCORTA 5"=0.0, "SCORTA 6"=0.0, "SCORTA 7"=0.0, "SCORTA 8"=0.0}, "statoAO_PLC out"={"Condensatori"=0.0, "Scorta 1"=0.0, "Scorta 2"=0.0}, "DO (bit)"={"Relè misura resistomat"=FALSE, "Misura res ramo 1"=FALSE, "Misura res ramo 2"=FALSE, "Misura res ramo 3"=FALSE, "Scelta banco 2"=FALSE, "Scala Torsiometro"=FALSE, "Ctrl torsiometro"=FALSE, "Select current mode"=FALSE, "Select Torque mode"=FALSE, "Select speed mode"=FALSE, "Watchdog"=FALSE, "Scorta"=FALSE, "Scorta 2"=FALSE, "Scorta 3"=FALSE, "Scorta 4"=FALSE, "Scorta 5"=FALSE, "Bench selection"=FALSE, "External alarm"=FALSE, "Enable external program"=FALSE, "Reset allarmi"=FALSE, "Start"=FALSE, "Stop"=FALSE, "Block"=FALSE, "Scorta 6"=FALSE}} ("USCITE PLC"), "DO (bit)"=w135) -> (w137:T19)
            n66 = Bundle By Name(cluster=T3 {"Message"="WRITE DO", "Data"=variant}, "Data"=w137) -> (w139:T3)
            n67 = Enqueue Element(queue=w136, element=w139) -> ()  [unwired: 2 in, 3 out]
          }
        }
      }
      frame #1 {
        n68 = Not Equal?(x=w144, y=w145) -> (x != y?=w143:bool)
        n69 = Or(x=w141, y=w143) -> (x .or. y?=w142:bool)
        n70 = case shown="True" w142 {
          tunnel: w147 -> [_ w149]
          tunnel: w146 -> [_ w148]
          frame False {
          }
          frame True {
            # "WRITE DO\nPLC 3"
            n71 = Bundle By Name(cluster=T20 {"AO (real) 2"={"SCORTA 1"=0.0, "SCORTA 2"=0.0, "SCORTA 3"=0.0, "SCORTA 4"=0.0, "SCORTA 5"=0.0, "SCORTA 6"=0.0, "SCORTA 7"=0.0, "SCORTA 8"=0.0}, "statoAO_PLC out"={"Rif velocità alimentatore"=0.0, "Scorta"=0.0, "Tipo Motore  keb"=0.0, "I nom keb"=0.0, "RPM nom keb"=0.0, "V nom keb"=0.0, "F nom keb"=0.0, "t rampa keb"=0.0}, "DO (bit)"={"Select linea Inverter"=FALSE, "Abilita sense wattmetro"=FALSE, "Bypass filtro LC"=FALSE, "Filtro LC"=FALSE, "Bypass trasformatore"=FALSE, "Trasformatore"=FALSE, "Abilita uscite variac"=FALSE, "Abilita linea 125 A"=FALSE, "Abilita linea 63 A"=FALSE, "Abilita linea 16 A"=FALSE, "Abilita Scrittura Dati Keb"=FALSE, "Abilita alimentatore"=FALSE, "Marcia alimentatore (1s)"=FALSE, "Stop alimentatore (1s)"=FALSE, "Senso rot mot prova"=FALSE, "Watchdog"=FALSE, "Aumenta tensione variac"=FALSE, "Diminuisci tensione variac "=FALSE, "Blocco elettroserrature"=FALSE, "Ripristino emergence"=FALSE, "Abilita ingresso variac"=FALSE, "Abilita ventilatore variac"=FALSE, "Reset Allarm"=FALSE, "Scorta 1"=FALSE, "Scorta 2"=FALSE, "Scorta 3"=FALSE, "Scorta 4"=FALSE, "Scorta 5"=FALSE, "Scorta 6"=FALSE, "Scorta 7"=FALSE, "Scorta 8"=FALSE, "Scorta 9"=FALSE, "Abilita collaudo"=FALSE, "Disabilita collaudo "=FALSE, "Scorta 10"=FALSE, "Scorta 11"=FALSE, "Scorta 12"=FALSE, "Scorta 13"=FALSE, "Scorta 14"=FALSE, "Scorta 15"=FALSE}} ("USCITE PLC"), "DO (bit)"=w148) -> (w153:T20)
            n72 = Bundle By Name(cluster=T3 {"Message"="WRITE DO", "Data"=variant}, "Data"=w153) -> (w151:T3)
            n73 = Enqueue Element(queue=w149, element=w151) -> ()  [unwired: 2 in, 3 out]
          }
        }
      }
    }
  }
  n74 = call "CALL_NI.vi"("banco"="banco", "simulazione"="simulazione") -> ()  [unwired: 10 in]
